vi "from string.vi"(8 "error in":errorcluster, 9 "data":string, 10 "version":string, 11 "Simple Sequencer TBM configuration in":refnum<class "Simple Sequencer TBM configuration.lvclass">) -> (0 "error out":errorcluster, 3 "Simple Sequencer TBM configuration out":refnum<class "Simple Sequencer TBM configuration.lvclass">)   [LabVIEW 2014, in "Simple Sequencer TBM configuration.lvclass"]
doc: "Provides an interface for loading a module configuration from a file or other serialized data source. It is recommended that all children of this class store data in two sets--data required for its own initialization, and any data required for parent initialization--and that each implementation uses the <b>Call Parent Method</b> primitive to de-serialize parent information. As a result, it is expected that every module configuration class calls <b>component configuration.lvclass:From String.vi</b>."
uses:
  Simple Sequencer TBM configuration.lvclass
  sequencer parent classes/action configuration parent/action configuration.lvclass
  Simple Sequencer TBM configuration.lvclass/Simple Sequencer TBM configuration.ctl
  sequencer parent classes/sequencer config parent/base TBM sequencer configuration.lvclass
  <vilib>/NI/Tag Bus Module Framework/module configuration/TBM module configuration.lvclass
  <vilib>/NI/Configuration Framework/serializable configuration/NISE_CEF_serializable configuration.lvclass
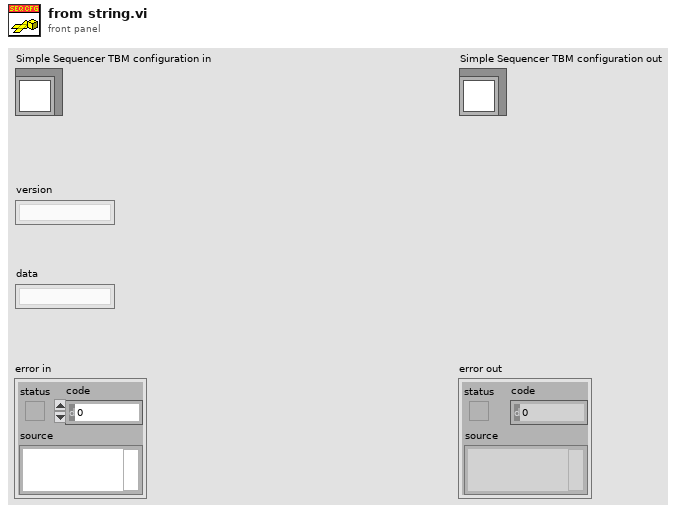
[diagram p1: front panel]
types:
  T1 = typedef "Simple Sequencer TBM configuration.lvclass/sequence definition.ctl" = cluster{"sequence name":string, "action configs":refnum<class "action configuration.lvclass">[]}
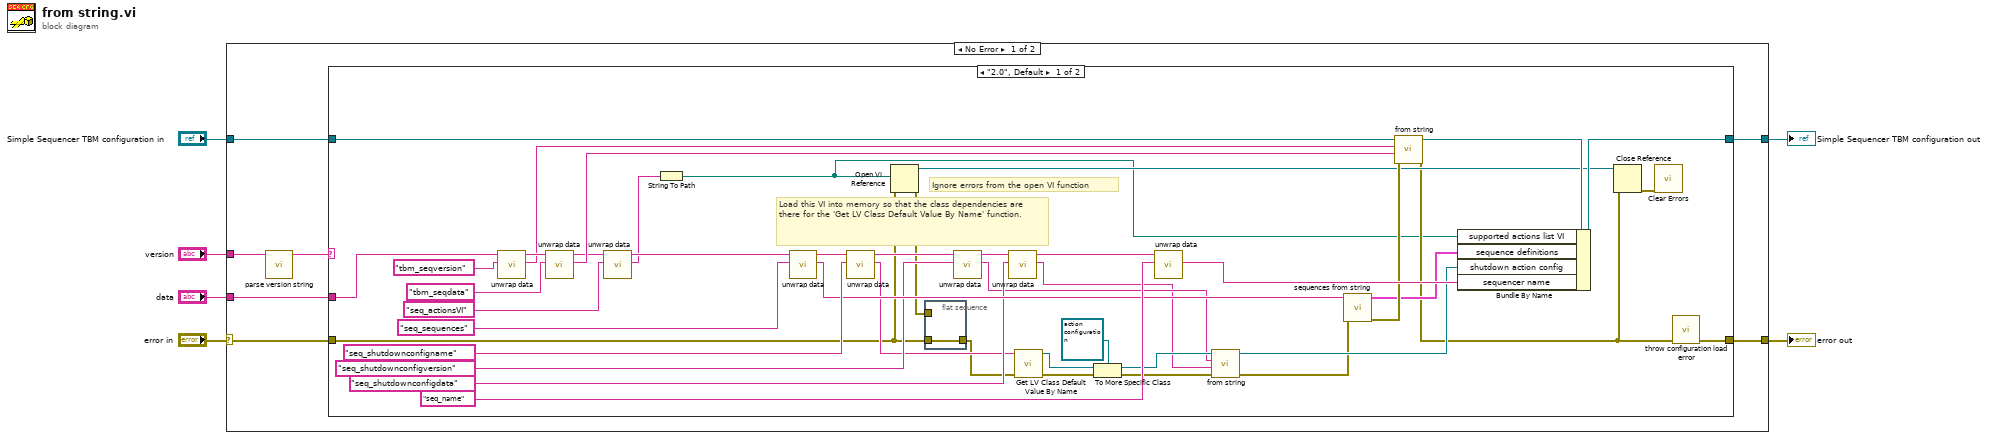
[diagram p0: block diagram]
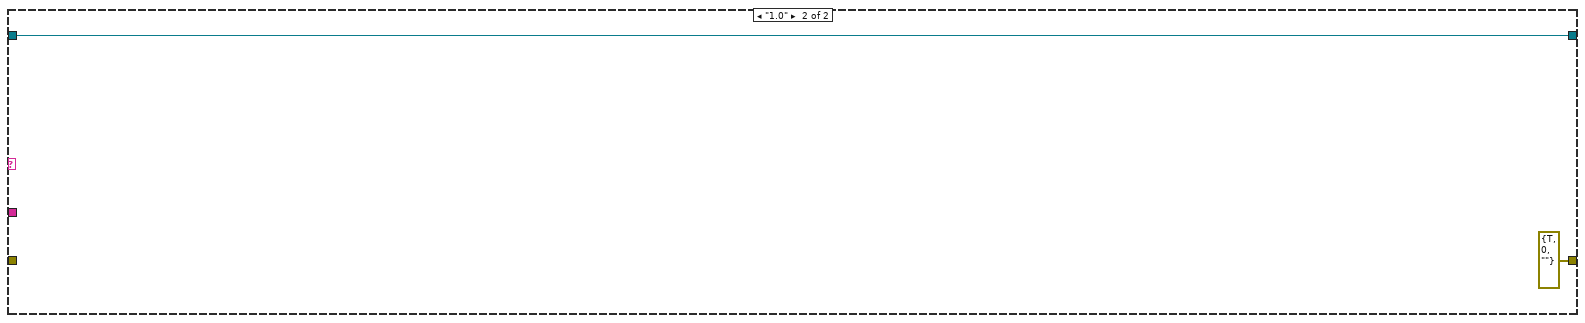
[diagram p2: hidden frame]
diagram:
  n1 = case shown="No Error" "error in" {
    selector: "error in" -> [w9 w62]
    tunnel: "data" -> [w13 _]
    tunnel: "Simple Sequencer TBM configuration in" -> [w12 w61]
    tunnel: [w11 w61] -> w5
    tunnel: [w10 w62] -> w4
    tunnel: "version" -> [w8 _]
    frame No Error {
      n2 = call <vilib>:"parse version string.vi"("full version"=w8) -> ("major.minor version"=w7:string)  [unwired: 7 in, 3 out]
      n3 = case shown="\"2.0\", Default" w7 {
        tunnel: w13 -> [w54 _]
        tunnel: w9 -> [w22 _]
        tunnel: w12 -> [w57 w60]
        tunnel: [w49 w60] -> w11
        tunnel: [w25 errorcluster {"status"=TRUE, "code"=0, "source"=""} ("error out")] -> w10
        frame "2.0", Default {
          # "Ignore errors from the open VI function"
          # "Load this VI into memory so that the class dependencies are there for the 'Get LV Class Default Value By Name' function."
          n4 = call <vilib>:"unwrap data.vi"("identifier"="tbm_seqversion" ("additional identifier"), "data to unwrap"=w54) -> ("unwrapped data"=w50:string, "remaining string"=w55:string)  [unwired: 8 in]
          n5 = call <vilib>:"unwrap data.vi"("identifier"="tbm_seqdata" ("additional identifier"), "data to unwrap"=w55) -> ("unwrapped data"=w52:string, "remaining string"=w18:string)  [unwired: 8 in]
          n6 = call <vilib>:"unwrap data.vi"("identifier"="seq_actionsVI", "data to unwrap"=w18) -> ("unwrapped data"=w15:string, "remaining string"=w17:string)  [unwired: 8 in]
          n7 = String To Path(string=w15) -> (path=w14:path)
          n8 = call <vilib>:"unwrap data.vi"("identifier"="seq_sequences", "data to unwrap"=w17) -> ("unwrapped data"=w43:string, "remaining string"=w48:string)  [unwired: 8 in]
          n9 = call <vilib>:"unwrap data.vi"("identifier"="seq_shutdownconfigname", "data to unwrap"=w48) -> ("unwrapped data"=w35:string, "remaining string"=w39:string)  [unwired: 8 in]
          n10 = Open VI Reference(vi path=w14, error in (no error)=w22) -> (vi reference=w24:refnum<vi>, error out=w23:errorcluster)  [unwired: 4 in]
          n11 = flat-sequence {
            tunnel: w23 -> [_]
            tunnel: w22 -> [w58]
            tunnel: [w58] -> w21
            frame #0 {
            }
          }
          n12 = call <vilib>:"unwrap data.vi"("identifier"="seq_shutdownconfigversion", "data to unwrap"=w39) -> ("unwrapped data"=w28:string, "remaining string"=w40:string)  [unwired: 8 in]
          n13 = call <vilib>:"unwrap data.vi"("identifier"="seq_shutdownconfigdata", "data to unwrap"=w40) -> ("unwrapped data"=w27:string, "remaining string"=w36:string)  [unwired: 8 in]
          n14 = call <vilib>:"Get LV Class Default Value By Name.vi"("error in (no error)"=w21, "class name"=w35) -> ("error out"=w34:errorcluster, "object"=w32:refnum<class>)  [unwired: 8 in]
          n15 = To More Specific Class(target class=refnum<class "action configuration.lvclass"> refnum ("shutdown action config"), reference=w32, error in=w34) -> (specific class reference=w31:refnum<class "action configuration.lvclass">, error out=w30:errorcluster)
          n16 = call <vilib>:"unwrap data.vi"("identifier"="seq_name", "data to unwrap"=w36) -> ("unwrapped data"=w45:string)  [unwired: 8 in, 1 out]
          n17 = call-dynamic "from string.vi"("error in"=w30, "data"=w27, "version"=w28, "configuration in"=w31) -> ("error out"=w26:errorcluster, "configuration out"=w29:refnum<class "action configuration.lvclass">)  [unwired: 6 in]
          n18 = call "sequences from string.vi"("error in (no error)"=w26, "data to unwrap"=w43) -> ("error out"=w42:errorcluster, "sequence definitions"=w41:T1[])  [unwired: 8 in]
          n19 = call-parent "from string.vi"("error in"=w42, "data"=w52, "version"=w50, "engine configuration in"=w57) -> ("error out"=w20:errorcluster, "engine configuration out"=w56:refnum<class "Simple Sequencer TBM configuration.lvclass">)  [unwired: 6 in]
          n20 = Bundle By Name(cluster=w56, "supported actions list VI"=w14, "sequence definitions"=w41, "shutdown action config"=w29, "sequencer name"=w45) -> (w49:refnum<class "Simple Sequencer TBM configuration.lvclass">)
          n21 = Close Reference(reference=w24, error in (no error)=w20) -> (error out=w19:errorcluster)
          n22 = call <vilib>:"Clear Errors.vi"("error in (no error)"=w19) -> ()  [unwired: 5 in, 2 out]
          n23 = call <vilib>:"throw configuration load error.vi"("error in"=w20) -> ("error out"=w25:errorcluster)  [unwired: 10 in]
        }
        frame "1.0" {
        }
      }
    }
    frame Error {
    }
  }
  "error out" <- w4
  "Simple Sequencer TBM configuration out" <- w5
